vi "AddOutToFile.vi"(8 "ErrorArray In":errorcluster[](array[cluster]), 11 "BusClass In":refnum<class "Bus.lvclass">) -> (0 "ErrorArray Out":errorcluster[](array[cluster]), 2 "clBroadcastEvents":T1, 3 "BusClass Out":refnum<class "Bus.lvclass">)   [LabVIEW 2017, in "Bus_class.lvlib" / "Bus.lvclass"]
uses:
  Bus.lvclass
  Modules/OutputToFileModule/Protected/Broadcasts/clBroadcastEvents.ctl
  Modules/OutputToFileModule/Private/clEventType.ctl
  Bus.lvclass/Bus.ctl
  <userlib>/NIST/ModuleAdminLib/ModuleAdmin/ModuleAdmin.lvclass
  Framework.lvlib
  <userlib>/NIST/NISTErrorLib/NISTErrorLib.lvlib
  Modules/OutputToFileModule/OutputToFileModule.lvlib
panel:
  # "If you want to add other Broadcast Events, open this typedef, copy an existing event and rename it to your event name.\n\nNext create an \"arg\" typedef for the  data and put it into PublicAPI/Arguments/Broadcasts\n\nAfter that, you will need to create a new roadcast vi in Protected/Broadcast.  Look at DidInit.vi or the reportError.vi as examples."
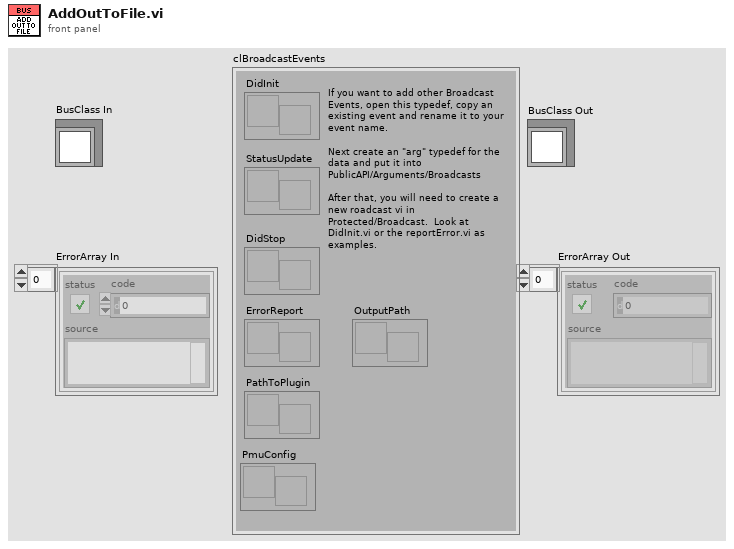
[diagram p1: front panel]
types:
  T1 = typedef "OutputToFileModule.lvlib/clBroadcastEvents.ctl" = cluster{"DidInit":refnum<user-event>, "StatusUpdate":refnum<user-event>, "ErrorReport":refnum<user-event>, "DidStop":refnum<user-event>, "PathToPlugin":refnum<user-event>, "PmuConfig":refnum<user-event>, "OutputPath":refnum<user-event>}
  T2 = typedef "Framework.lvlib/clFrameworkData.ctl" = cluster{"EvtINIFilePaths":path[], "BusClassInstances":refnum<class "Bus.lvclass">[], "PmuImpairINIFilePaths":path[], "FlagImpairINIFilePaths":path[], "NetImpairINIFilePaths":path[], "OutputToFileINIFilePaths":path[], "AppINIFilePaths":path[], "AppModuleID":i32, "OutputToFileID":i32}
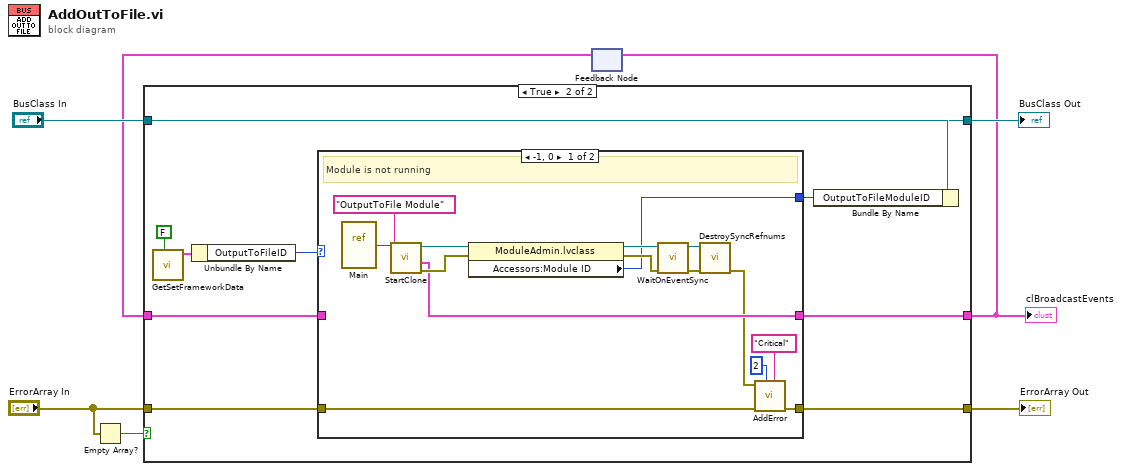
[diagram p0: block diagram]
diagram:
  n1 = Empty Array?(array="ErrorArray In") -> (empty?=w7:bool)
  n2 = feedback #1() -> (w1:T1)  [unwired: 1 in]
  n3 = case shown="True" w7 {
    tunnel: "ErrorArray In" -> [w10 w17]
    tunnel: [w10 w16] -> w5
    tunnel: "BusClass In" -> [w9 w13]
    tunnel: [w9 w12] -> w3
    tunnel: [w8 w15] -> w2
    tunnel: w1 -> [w8 w14]
    frame False {
    }
    frame True {
      n4 = call "GetSetFrameworkData.vi"("Set (F)"=FALSE) -> ("clFrameworkData Out"=w18:T2)  [unwired: 10 in]
      n5 = Unbundle By Name(w18) -> ("OutputToFileID"=w19:i32)
      n6 = case shown="-1, 0" w19 {
        selector: w19 -> [_ w36]
        tunnel: w17 -> [w27 w38]
        tunnel: [w24 w38] -> w16
        tunnel: [w23 w37] -> w15
        tunnel: w14 -> [_ w37]
        tunnel: [w21 w36] -> w11
        frame -1, 0 {
          # "Module is not running"
          n7 = vi-ref "Main.vi"() -> (w35:refnum<vi>)
          n8 = call "StartClone.vi"("ModuleName"="OutputToFile Module", "VI Refnum"=w35) -> ("error out"=w32:errorcluster, "clBroadcastEvents"=w23:T1, "ModuleAdmin"=w33:refnum<class "ModuleAdmin.lvclass">)  [unwired: 7 in]
          n9 = property class="ModuleAdmin.lvclass"(reference=w33, error in=w32) -> (reference out=w31:refnum<class "ModuleAdmin.lvclass">, error out=w28:errorcluster, "Accessors:Module ID"=w21:i32)
          n10 = call <userlib>:"WaitOnEventSync.vi"("error in (no error)"=w28, "ModuleAdmin"=w31) -> ("error out"=w30:errorcluster, "ModuleAdmin"=w29:refnum<class "ModuleAdmin.lvclass">)  [unwired: 8 in]
          n11 = call <userlib>:"DestroySyncRefnums.vi"("error in (no error)"=w30, "ModuleAdmin"=w29) -> ("error out"=w22:errorcluster)  [unwired: 9 in]
          n12 = call <userlib>:"AddError.vi"("Severity"="Critical", "Priority"=u8 2, "ErrorArray"=w27, "error in (no error)"=w22) -> ("ErrorArray"=w24:errorcluster[])  [unwired: 6 in, 1 out]
        }
        frame 1, Default {
          # "Module is already running"
        }
      }
      n13 = Bundle By Name(cluster=w13, "OutputToFileModuleID"=w11) -> (w12:refnum<class "Bus.lvclass">)
    }
  }
  "ErrorArray Out" <- w5
  "BusClass Out" <- w3
  "clBroadcastEvents" <- w2
  n14 = feedback-in #1(w2) -> ()
